vi "fp5touch.vi"   [LabVIEW 2016]
uses:
  <vilib>/NXT/Block Support/NXT_OutputPort.ctl
  <vilib>/NXT/Block Support/NXT_InputPort.ctl
  <vilib>/NXT/NXTIO Xnodes/NXTIONodeSubVIs/LEGOResetMotors.vi
  <vilib>/NXT/Dual Mode Library/Sensors/Touch_Pressed.vi
  <vilib>/NXT/Dual Mode Library/Sensors/EV3_Color_Reflect.vi
  <vilib>/NXT/NXTIO Xnodes/NXTIONodeSubVIs/NXTMoveMotors.vi
  <vilib>/NXT/NXTIO Xnodes/NXTIONodeSubVIs/NXTMotorRunDistance.vi
  <vilib>/NXT/NXTIO Xnodes/NXTIONodeSubVIs/NXTStopMotors.vi
  <vilib>/NXT/Dual Mode Library/Sound/PlayAsharp.vi
  <vilib>/NXT/Dual Mode Library/Sound/PlayC.vi
  <vilib>/NXT/Subs/LVHSConnector.ctl
  <vilib>/NXT/NXTIO Xnodes/AddressXNode/NXTIOAddress.xnode
  <vilib>/NXT/NXTIO Xnodes/NXTIOXNode/NXTIO.xnode
  <vilib>/NXT/LegoClasses/BrickReference/BrickReference.lvclass
types:
  T1 = typedef "NXT_OutputPort.ctl" = u8
  T2 = typedef "NXT_InputPort.ctl" = u32
  T3 = typedef "LVHSConnector.ctl" = refnum<class "BrickReference.lvclass">
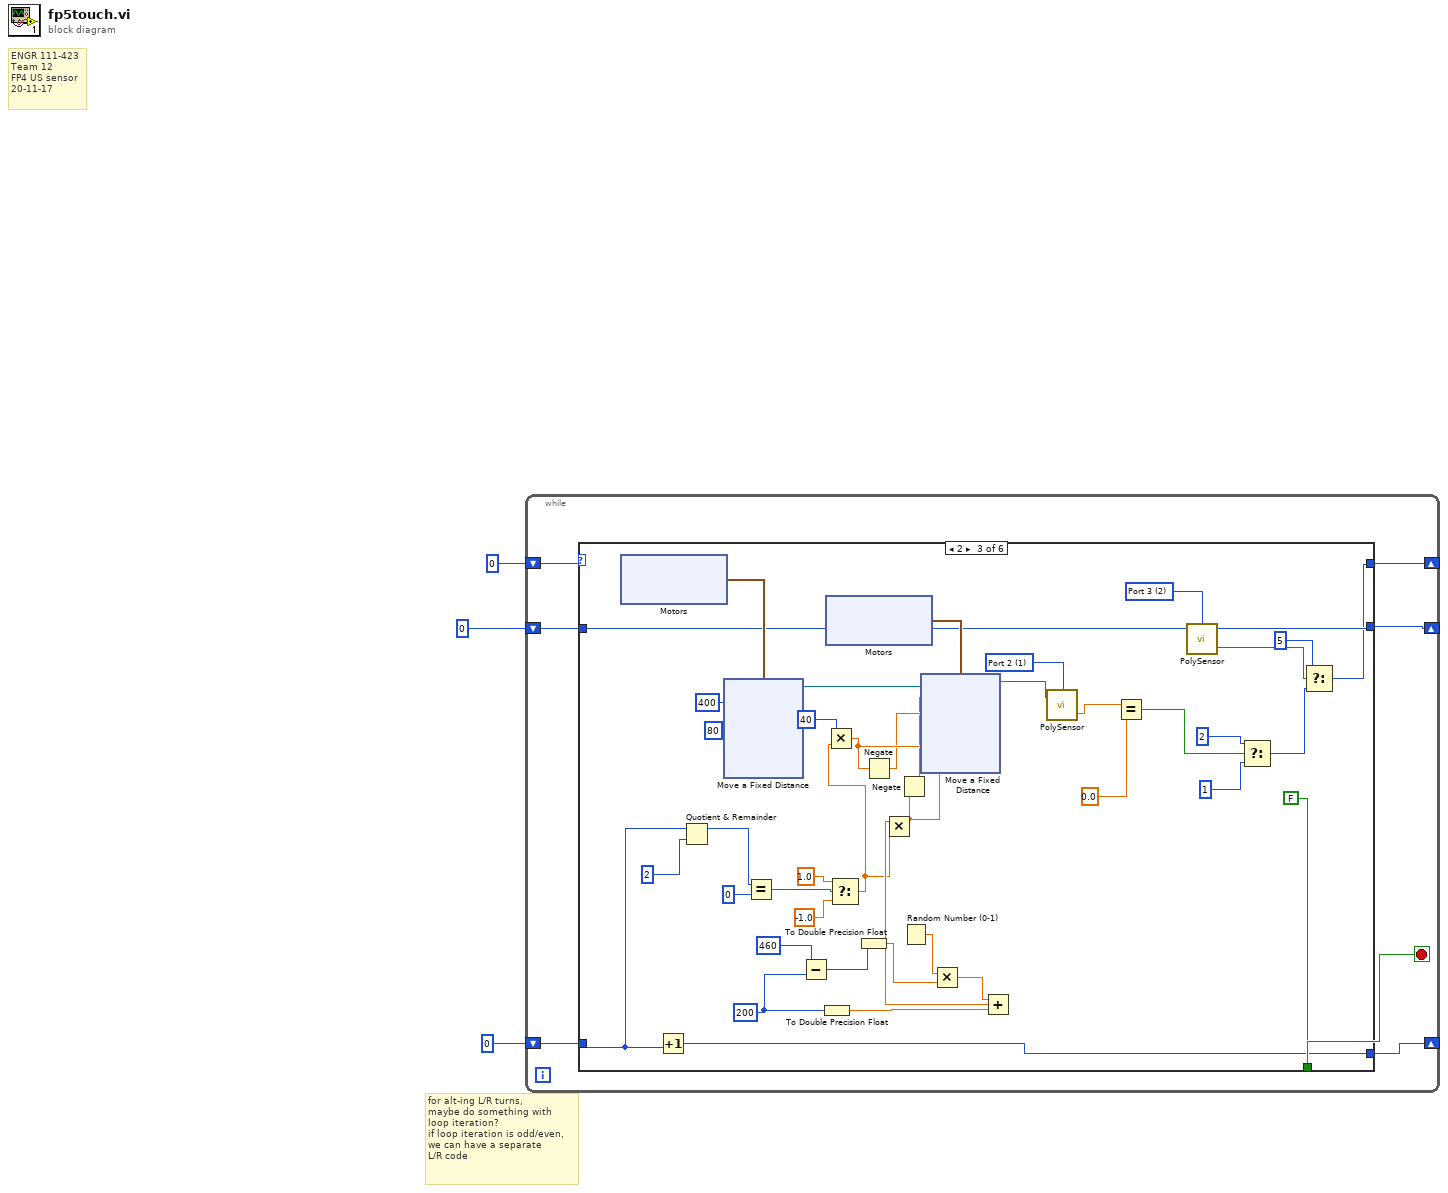
[diagram p0: block diagram]
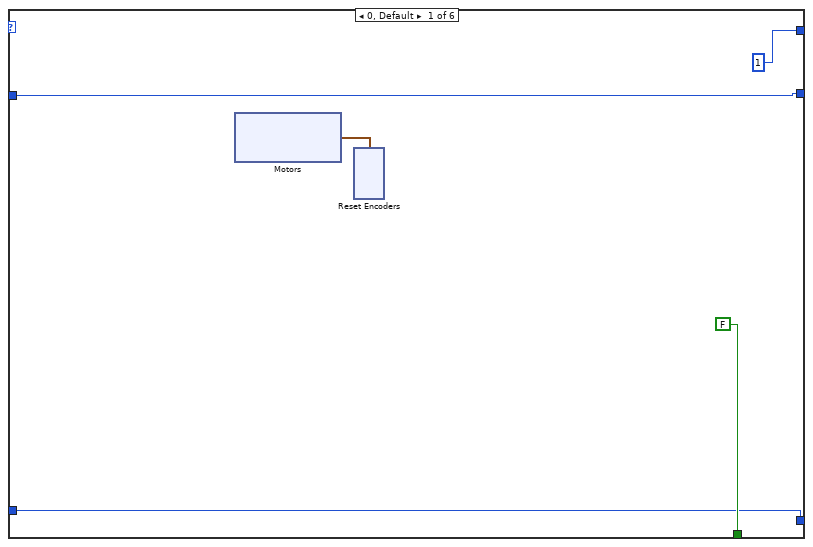
[diagram p2: hidden frame]
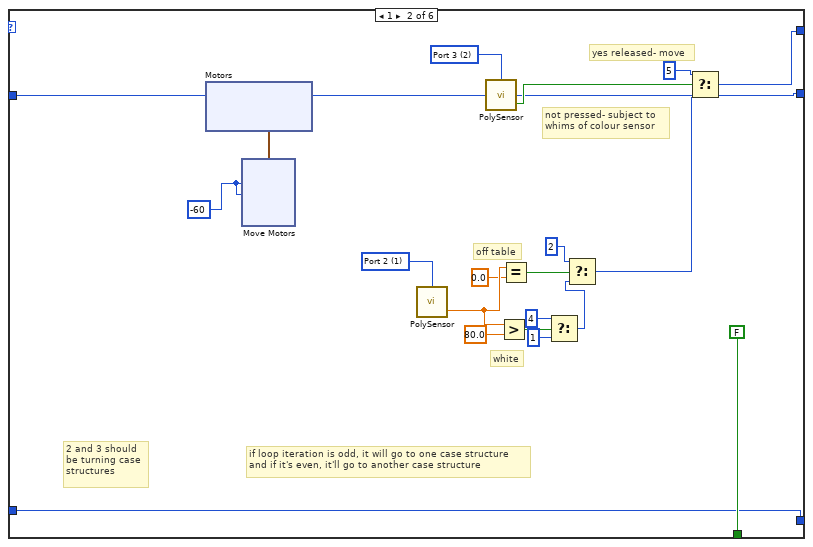
[diagram p3: hidden frame]
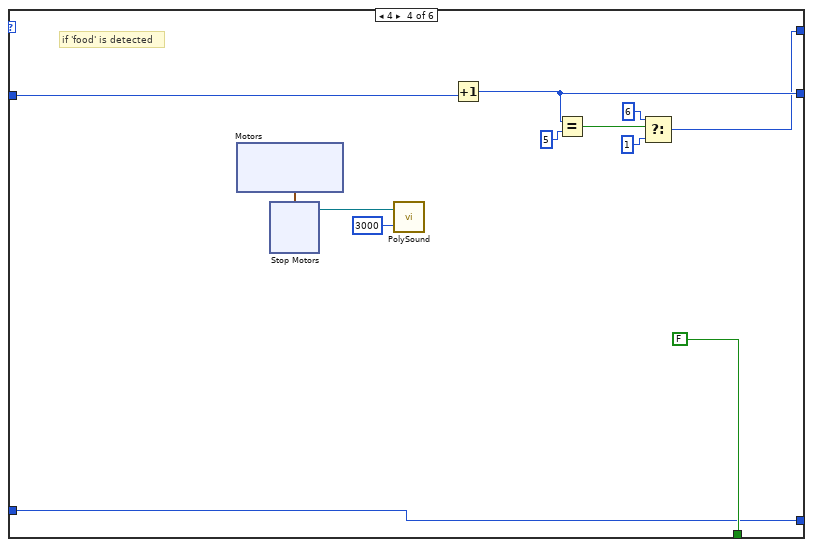
[diagram p4: hidden frame]
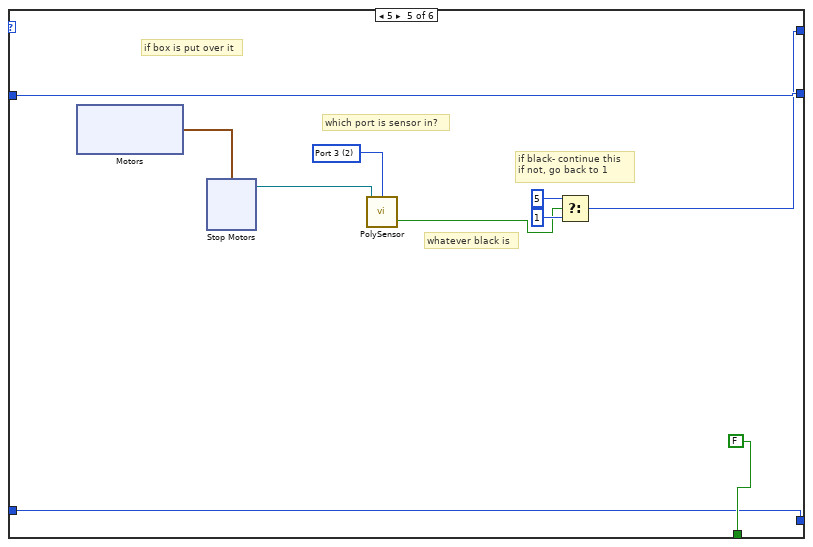
[diagram p5: hidden frame]
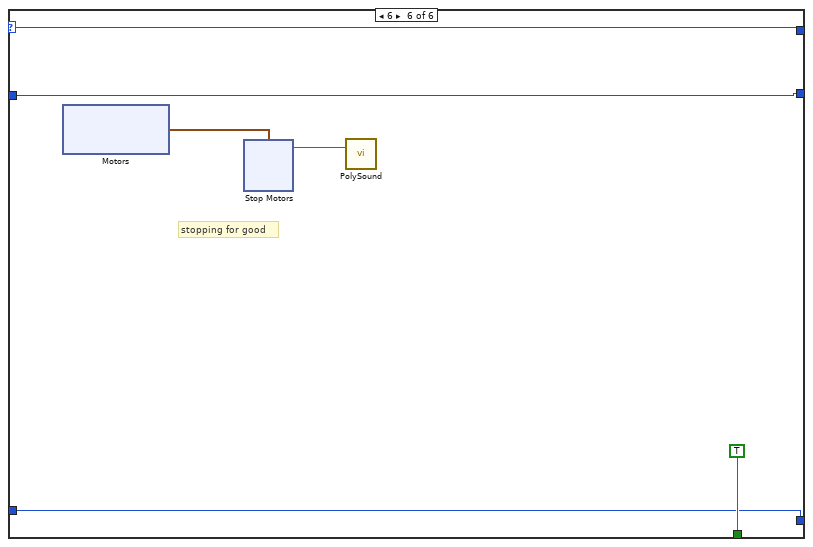
[diagram p6: hidden frame]
diagram:
  # "for alt-ing L/R turns,\nmaybe do something with\nloop iteration?\nif loop iteration is odd/even,\nwe can have a separate\nL/R code"
  # "ENGR 111-423\nTeam 12\nFP4 US sensor\n20-11-17"
  n1 = while {
    shift-right: [w8] -> _
    shift-left: 0 -> [w10]
    shift-right: [w6] -> _
    shift-left: 0 -> [w7]
    shift-right: [w4] -> _
    shift-left: 0 -> [w5]
    stop <- w9 stop-if-true
    n2 = case shown="2" w10 {
      selector: w10 -> [_ _ _ _ _ w155]
      tunnel: [FALSE FALSE FALSE FALSE FALSE TRUE] -> w9
      tunnel: [1 w29 w64 w118 w135 w155] -> w8
      tunnel: w7 -> [w12 w25 w65 w125 w140 w152]
      tunnel: [w12 w25 w65 w122 w140 w152] -> w6
      tunnel: w5 -> [w11 w21 w51 w117 w136 w151]
      tunnel: [w11 w21 w52 w117 w136 w151] -> w4
      frame 0, Default {
        n3 = xnode "Motors"() -> ("Motor"=w13:cluster{"Port":T1, "Port":T1})
        n4 = xnode "Reset Encoders"("Motors"=w13) -> ()  [unwired: 1 in, 1 out]
      }
      frame 1 {
        w30 = T2 1 items=["Port 1", "Port 2", "Port 3", "Port 4"] ("Port (Port 1)")
        w38 = T2 2 items=["Port 1", "Port 2", "Port 3", "Port 4"] ("Port (Port 1)")
        w39 = -60 ("Distance 1")
        # "white"
        # "off table"
        # "2 and 3 should\nbe turning case\nstructures"
        # "if loop iteration is odd, it will go to one case structure\nand if it's even, it'll go to another case structure"
        # "not pressed- subject to\nwhims of colour sensor"
        # "yes released- move"
        n5 = xnode "Motors"() -> ("Motor"=w40:cluster{"Port":T1, "Port":T1})
        n6 = xnode "Move Motors"("Power/Speed 2"=w39, "Power/Speed 1"=w39, "Motors"=w40) -> ()  [unwired: 1 in, 1 out]
        n7 = call-poly <vilib>:"PolySensor.vi"("Port (Port 1)"=w30) -> ("Scaled Value"=w31:sgl)  [unwired: 2 in, 1 out]
        n8 = call-poly <vilib>:"PolySensor.vi"("Port (Port 1)"=w38) -> ("Yes / No"=w37:bool)  [unwired: 2 in, 1 out]
        n9 = Greater?(x=w31, y=sgl 80.0) -> (0:w35:bool)
        n10 = Equal?(x=w31, y=sgl 0.0) -> (x = y?=w33:bool)
        n11 = Select(t=i16 4, s=w35, f=i16 1) -> (s? t:f=w27:i16)
        n12 = Select(t=2, s=w33, f=w27) -> (s? t:f=w22:i32)
        n13 = Select(t=i16 5, s=w37, f=w22) -> (s? t:f=w29:i32)
      }
      frame 2 {
        w61 = 200
        w78 = 80 ("Distance 1")
        w79 = 400 ("Distance 1")
        w83 = T2 1 items=["Port 1", "Port 2", "Port 3", "Port 4"] ("Port (Port 1)")
        w85 = T2 2 items=["Port 1", "Port 2", "Port 3", "Port 4"] ("Port (Port 1)")
        n14 = xnode "Motors"() -> ("Motor"=w80:cluster{"Port":T1, "Port":T1})
        n15 = Increment(x=w51) -> (x+1=w52:i32)
        n16 = Quotient & Remainder(x=w51, y=2) -> (x-y*floor(x/y)=w72:i32)  [unwired: 1 out]
        n17 = xnode "Move a Fixed Distance"("Speed 2"=w78, "Speed 1"=w78, "Distance 2"=w79, "Distance 1"=w79, "Motors"=w80) -> ("NXT/EV3"=w53:T3)  [unwired: 1 in]
        n18 = Equal?(x=w72, y=0) -> (x = y?=w70:bool)
        n19 = Subtract(x=460, y=w61) -> (x-y=w62:i32)
        n20 = To Double Precision Float(number=w61) -> (double precision float=w57:dbl)
        n21 = xnode "Motors"() -> ("Motor"=w81:cluster{"Port":T1, "Port":T1})
        n22 = Select(t=1.0, s=w70, f=-1.0) -> (s? t:f=w55:dbl)
        n23 = Multiply(x=40 ("Distance 1"), y=w55) -> (x*y=w75:dbl)
        n24 = To Double Precision Float(number=w62) -> (double precision float=w60:dbl)
        n25 = Negate(x=w75) -> (-x=w74:dbl)
        n26 = Random Number (0-1)() -> (number: 0 to 1=w59:dbl)
        n27 = Multiply(x=w59, y=w60) -> (x*y=w58:dbl)
        n28 = Add(x=w58, y=w57) -> (x+y=w56:dbl)
        n29 = Multiply(x=w56, y=w55) -> (x*y=w54:dbl)
        n30 = Negate(x=w54) -> (-x=w67:dbl)
        n31 = xnode "Move a Fixed Distance"("Speed 2"=w75, "Speed 1"=w74, "Distance 2"=w54, "Distance 1"=w67, "Motors"=w81, "NXT/EV3"=w53) -> ("NXT/EV3"=w50:T3)
        n32 = call-poly <vilib>:"PolySensor.vi"("NXT/EV3"=w50, "Port (Port 1)"=w83) -> ("Scaled Value"=w82:sgl)  [unwired: 1 in, 1 out]
        n33 = Equal?(x=w82, y=0.0) -> (x = y?=w86:bool)
        n34 = call-poly <vilib>:"PolySensor.vi"("Port (Port 1)"=w85) -> ("Yes / No"=w84:bool)  [unwired: 2 in, 1 out]
        n35 = Select(t=2, s=w86, f=1) -> (s? t:f=w89:i32)
        n36 = Select(t=5, s=w84, f=w89) -> (s? t:f=w64:i32)
      }
      frame 4 {
        # "if 'food' is detected"
        n37 = xnode "Motors"() -> ("Motor"=w127:cluster{"Port":T1, "Port":T1})
        n38 = xnode "Stop Motors"("Motors"=w127) -> ("NXT/EV3"=w128:T3)  [unwired: 1 in]
        n39 = call-poly <vilib>:"PolySound.vi"("Duration (500 ms)"=u16 3000, "NXT/EV3"=w128) -> ()  [unwired: 2 in, 1 out]
        n40 = Increment(x=w125) -> (x+1=w122:i32)
        n41 = Equal?(x=w122, y=5) -> (x = y?=w123:bool)
        n42 = Select(t=6, s=w123, f=1) -> (s? t:f=w118:i32)
      }
      frame 5 {
        w138 = T2 2 items=["Port 1", "Port 2", "Port 3", "Port 4"] ("Port (Port 1)")
        # "if black- continue this\nif not, go back to 1"
        # "whatever black is"
        # "which port is sensor in?"
        # "if box is put over it"
        n43 = xnode "Motors"() -> ("Motor"=w144:cluster{"Port":T1, "Port":T1})
        n44 = xnode "Stop Motors"("Motors"=w144) -> ("NXT/EV3"=w139:T3)  [unwired: 1 in]
        n45 = call-poly <vilib>:"PolySensor.vi"("NXT/EV3"=w139, "Port (Port 1)"=w138) -> ("Yes / No"=w137:bool)  [unwired: 1 in, 1 out]
        n46 = Select(t=i16 5, s=w137, f=i16 1) -> (s? t:f=w135:i16)
      }
      frame 6 {
        # "stopping for good"
        n47 = xnode "Motors"() -> ("Motor"=w156:cluster{"Port":T1, "Port":T1})
        n48 = xnode "Stop Motors"("Motors"=w156) -> ("NXT/EV3"=w153:T3)  [unwired: 1 in]
        n49 = call-poly <vilib>:"PolySound.vi"("NXT/EV3"=w153) -> ()  [unwired: 3 in, 1 out]
      }
    }
  }
